vi "Destroy User Event - ConnectionEvent.vi"(8 "error in (no error)":errorcluster, 11 "user event out":refnum<user-event>) -> (0 "error out":errorcluster)   [LabVIEW 2022 SP3, in "User Event - ConnectionEvent.lvlib"]
doc: "Destroy the user event, even if there is an incoming error."
uses:
  User Event - ConnectionEvent.lvlib
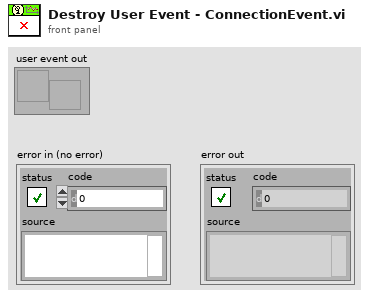
[diagram p1: front panel]
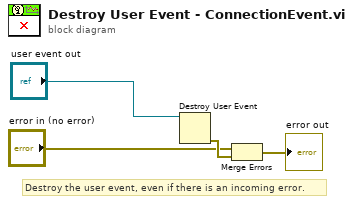
[diagram p0: block diagram]
diagram:
  # "Destroy the user event, even if there is an incoming error."
  n1 = Destroy User Event(user event="user event out") -> (error out=w4:errorcluster)  [unwired: 1 in]
  n2 = Merge Errors("error in (no error)", w4) -> (→"error out":errorcluster)
